vi "Target Data Listeners.vi"(8 "error in":errorcluster, 10 "set? (F)":bool, 11 "Listener":T1) -> (0 "error out":errorcluster, 3 "Listeners":T1[](array[typedef]))   [LabVIEW 2016, in "Vision Server.lvclass"]
uses:
  Vision Server.lvclass
  typedef/Target Listener Queue.ctl
  typedef/Target Message JSON.ctl
  typedef/Target Vector.ctl
panel:
  # "List of queues to publish target data"
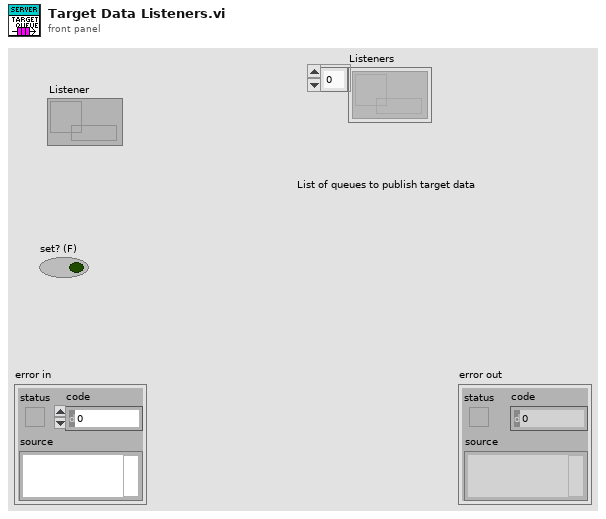
[diagram p1: front panel]
types:
  T1 = typedef "Vision Server.lvclass/Target Listener Queue.ctl" = refnum<queue>
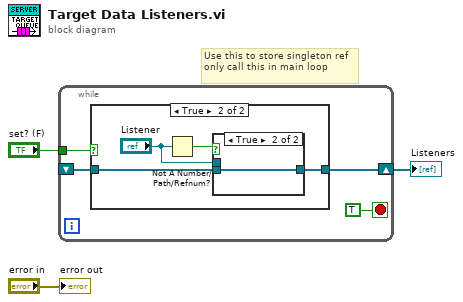
[diagram p0: block diagram]
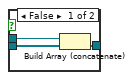
[diagram p3: hidden frame]
diagram:
  # "Use this to store singleton ref only call this in main loop"
  n1 = while {
    tunnel: "set? (F)" -> [w7]
    shift-right: [w6] -> w1
    shift-left: _ -> [w5]
    stop <- TRUE stop-if-true
    n2 = case shown="True" w7 {
      tunnel: [w8 w12] -> w6
      tunnel: w5 -> [w8 w11]
      frame False {
      }
      frame True {
        n3 = Not A Number/Path/Refnum?(number/path/refnum="Listener") -> (NaN/Path/Refnum?=w10:bool)
        n4 = case shown="True" w10 {
          tunnel: [w15 w16] -> w12
          tunnel: w11 -> [w14 w16]
          tunnel: "Listener" -> [w13 _]
          frame False {
            n5 = Build Array (concatenate)(w13, w14) -> (w15:T1[])
          }
          frame True {
          }
        }
      }
    }
  }
  "Listeners" <- w1
  "error out" <- "error in"
